vi "Build Exit Next Frame Check.vi"(7 "Virtual Memory Unit in":refnum<class "Virtual Memory Unit.lvclass">, 8 "error in (no error)":errorcluster, 10 "Starting Address":u16 format="%04x", 11 "Major Frame in":refnum<class "Major Frame.lvclass">) -> (0 "error out":errorcluster, 2 "Next Available Address":u16 format="%04x", 3 "Major Frame out":refnum<class "Major Frame.lvclass">, 5 "Virtual Memory Unit out":refnum<class "Virtual Memory Unit.lvclass">)   [LabVIEW 2016, in "BCI-1553 API.lvlib" / "Major Frame.lvclass"]
doc: "Resets the frame timer (which is used for determining if we have time for async stuff and more). Afterwards, we leave this minor frame check subroutine and advance to the next minor frame."
uses:
  Major Frame.lvclass
  TypeDefs/BC Condition Codes.ctl
  BCI-1553 API.lvlib
  TypeDefs/BC Op Codes - Verbose.ctl
  Dependencies/Virtual Memory Unit/Virtual Memory Unit.lvclass
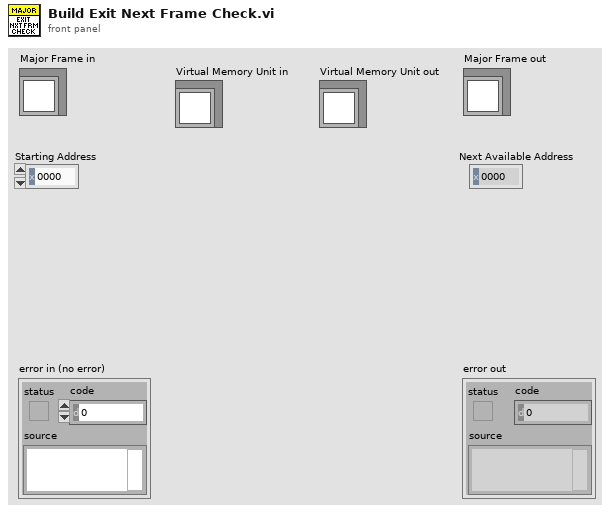
[diagram p1: front panel]
types:
  T1 = typedef "BCI-1553 API.lvlib/BC Op Codes - Verbose.ctl" = enum16{"EXECUTE MSG", "EXECUTE MSG GO", "JUMP", "CALL SUBROUTINE", "RETURN", "INTERRUPT REQUEST", "HALT", "DELAY", "WAIT FRAME TIMER = 0", "COMPARE FRAME TIMER", "COMPARE MSG TIMER", "LOAD TIME TAG CTR", "LOAD TIME TAG CTR HI", "LOAD FRAME TIMER", "START FRAME TIMER", "PUSH TIME TAG COUNT", "PUSH TIME TAG COUNT HI", "PUSH TIME TAG COUNT BOTH", "PUSH BLOCK STATUS WORD", "PUSH CURRENT VALUE", "PUSH INDIRECT", "WAIT EXT TRIGGER", "EXECUTE AND FLIP", "EXECUTE, FLIP, GO", "WRITE VALUE TO WMI", "WRITE VALUE TO MEM", "DECREMENT RAM, SKIP", "FLAG"}
  T2 = typedef "BCI-1553 API.lvlib/BC Condition Codes.ctl" = enum16{"GP0 == 1 || LT", "GP1 == 1 || NE", "GP2 == 1", "GP3 == 1", "GP4 == 1", "GP5 == 1", "GP6 == 1", "GP7 == 1", "NORESP", "FMTERR", "GOODBLOCK", "MSKSTATSET", "BADMSG", "1RETRY", "2RETRY", "ALWAYS"}
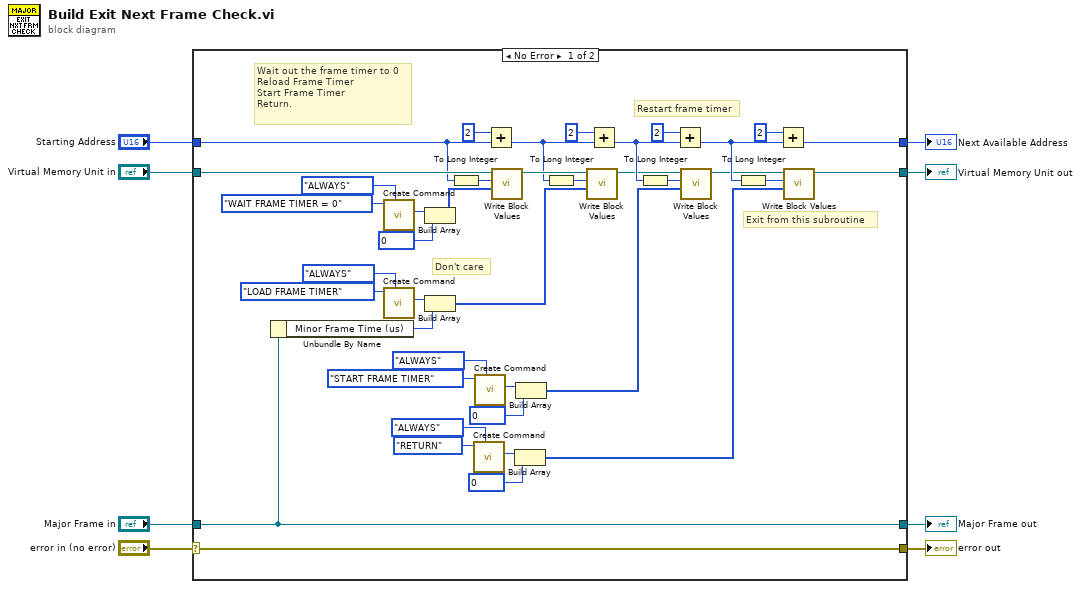
[diagram p0: block diagram]
diagram:
  n1 = case shown="No Error" "error in (no error)" {
    selector: "error in (no error)" -> [w48 w52]
    tunnel: [w48 w52] -> w7
    tunnel: [w13 w51] -> w5
    tunnel: "Major Frame in" -> [w13 w51]
    tunnel: "Virtual Memory Unit in" -> [w12 w49]
    tunnel: "Starting Address" -> [w11 w50]
    tunnel: [w10 w50] -> w2
    tunnel: [w9 w49] -> w1
    frame No Error {
      # "Exit from this subroutine"
      # "Restart frame timer"
      # "Don't care"
      # "Wait out the frame timer to 0\nReload Frame Timer\nStart Frame Timer\nReturn."
      n2 = Unbundle By Name(w13) -> ("Minor Frame Time (us)"=w29:u16)
      n3 = call "Create Command.vi"("Condition"=BC_Condition_Codes."ALWAYS", "Op Code"=BC_Op_Codes_-_Verbose."WAIT FRAME TIMER = 0") -> ("Instruction"=w26:u16)  [unwired: 8 in, 1 out]
      n4 = call "Create Command.vi"("Condition"=BC_Condition_Codes."ALWAYS", "Op Code"=BC_Op_Codes_-_Verbose."LOAD FRAME TIMER") -> ("Instruction"=w20:u16)  [unwired: 8 in, 1 out]
      n5 = Build Array(w26, u16 0 ("element")) -> (w24:u16[])
      n6 = Build Array(w20, w29) -> (w21:u16[])
      n7 = To Long Integer(number=w11) -> (32bit integer=w23:i32)
      n8 = call "Create Command.vi"("Condition"=BC_Condition_Codes."ALWAYS", "Op Code"=BC_Op_Codes_-_Verbose."RETURN") -> ("Instruction"=w38:u16)  [unwired: 8 in, 1 out]
      n9 = call "Create Command.vi"("Condition"=BC_Condition_Codes."ALWAYS", "Op Code"=BC_Op_Codes_-_Verbose."START FRAME TIMER") -> ("Instruction"=w32:u16)  [unwired: 8 in, 1 out]
      n10 = Add(x=u16 2, y=w11) -> (x+y=w16:u16)
      n11 = call "Write Block Values.vi"("Write Block"=w24, "Start Index"=w23, "Virtual Memory Unit in"=w12) -> ("Virtual Memory Unit out"=w17:refnum<class "Virtual Memory Unit.lvclass">)  [unwired: 7 in, 1 out]
      n12 = Build Array(w38, u16 0 ("element")) -> (w45:u16[])
      n13 = Build Array(w32, u16 0 ("element")) -> (w34:u16[])
      n14 = To Long Integer(number=w16) -> (32bit integer=w22:i32)
      n15 = call "Write Block Values.vi"("Write Block"=w21, "Start Index"=w22, "Virtual Memory Unit in"=w17) -> ("Virtual Memory Unit out"=w35:refnum<class "Virtual Memory Unit.lvclass">)  [unwired: 7 in, 1 out]
      n16 = Add(x=u16 2, y=w16) -> (x+y=w36:u16)
      n17 = To Long Integer(number=w36) -> (32bit integer=w46:i32)
      n18 = Add(x=u16 2, y=w36) -> (x+y=w44:u16)
      n19 = call "Write Block Values.vi"("Write Block"=w34, "Start Index"=w46, "Virtual Memory Unit in"=w35) -> ("Virtual Memory Unit out"=w43:refnum<class "Virtual Memory Unit.lvclass">)  [unwired: 7 in, 1 out]
      n20 = To Long Integer(number=w44) -> (32bit integer=w42:i32)
      n21 = Add(x=u16 2, y=w44) -> (x+y=w10:u16)
      n22 = call "Write Block Values.vi"("Write Block"=w45, "Start Index"=w42, "Virtual Memory Unit in"=w43) -> ("Virtual Memory Unit out"=w9:refnum<class "Virtual Memory Unit.lvclass">)  [unwired: 7 in, 1 out]
    }
    frame Error {
    }
  }
  "error out" <- w7
  "Major Frame out" <- w5
  "Next Available Address" <- w2
  "Virtual Memory Unit out" <- w1
